vi "CreateValveCases.vi"(9 "Ctr Water Valve":string, 10 "Ctr Odor Valve":string, 11 "Valve In":string) -> (3 "Case":enum16{"Odors", "Controls", "Water Mix"}(ring))   [LabVIEW 2016]
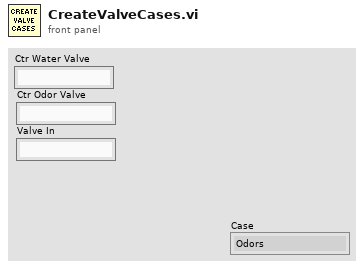
[diagram p1: front panel]
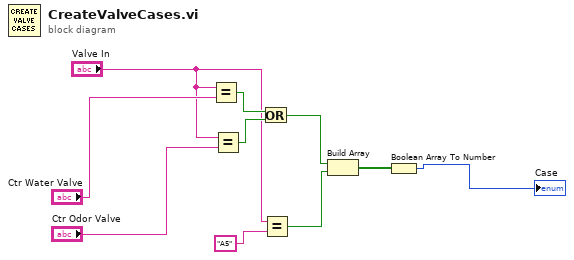
[diagram p0: block diagram]
diagram:
  n1 = Equal?(x="Valve In", y="Ctr Water Valve") -> (x = y?=w7:bool)
  n2 = Equal?(x="Valve In", y="Ctr Odor Valve") -> (x = y?=w8:bool)
  n3 = Or(x=w7, y=w8) -> (x .or. y?=w3:bool)
  n4 = Equal?(x="Valve In", y="A5") -> (x = y?=w4:bool)
  n5 = Build Array(w3, w4) -> (w2:bool[])
  n6 = Boolean Array To Number(Boolean array=w2) -> (number=→"Case":u32)
